vi "serialization test.vi"() -> (0 "no error":errorcluster, 1 "name ok":bool, 2 "serOK":bool, 3 "class identical":bool, 4 "keys ok":bool, 5 "version ok":bool)   [LabVIEW 2025, in "NISE_CEF_Tests.lvlib"]
uses:
  NISE_CEF_Tests.lvlib
  Trunk/Configuration Framework/serializable configuration/NISE_CEF_serializable configuration.lvclass
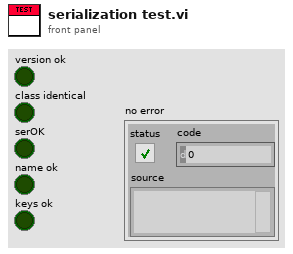
[diagram p1: front panel]
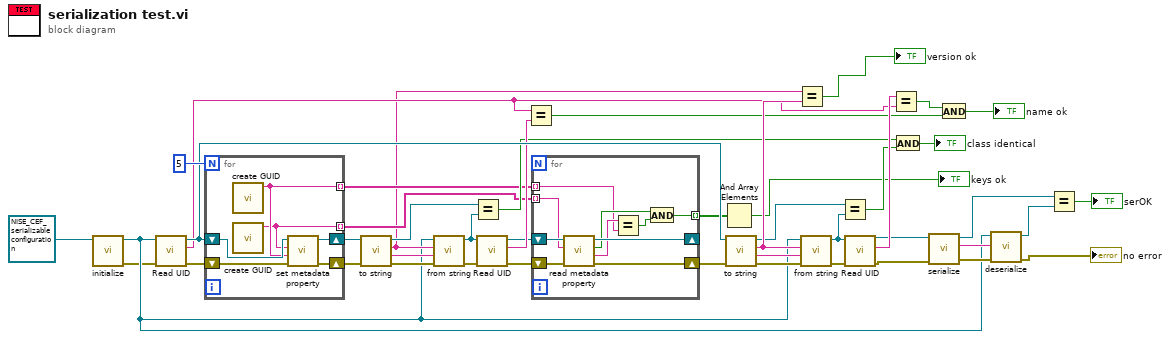
[diagram p0: block diagram]
diagram:
  n1 = call "initialize.vi"("configuration in"=refnum<class "NISE_CEF_serializable configuration.lvclass"> refnum ("configuration")) -> ("error out"=w1:errorcluster, "configuration out"=w2:refnum<class "NISE_CEF_serializable configuration.lvclass">)  [unwired: 8 in, 1 out]
  n2 = call "Read UID.vi"("error in"=w1, "configuration in"=w2) -> ("error out"=w38:errorcluster, "instance id"=w30:string, "configuration out"=w39:refnum<class "NISE_CEF_serializable configuration.lvclass">)  [unwired: 7 in]
  n3 = for {
    N: 5 -> [_]
    shift-right: [w50] -> w29
    shift-left: w39 -> [w51]
    shift-right: [w49] -> w35
    shift-left: w38 -> [w48]
    tunnel: [w47] -> w19 mode=indexing
    tunnel: [w46] -> w20 mode=indexing
    n4 = call "create GUID.vi"() -> ("uuid"=w47:string)  [unwired: 10 in, 1 out]
    n5 = call "create GUID.vi"() -> ("uuid"=w46:string)  [unwired: 10 in, 1 out]
    n6 = call "set metadata property.vi"("error in"=w48, "value"=w47, "key"=w46, "configuration in"=w51) -> ("error out"=w49:errorcluster, "configuration out"=w50:refnum<class "NISE_CEF_serializable configuration.lvclass">)  [unwired: 6 in]
  }
  n7 = call-dynamic "to string.vi"("error in"=w35, "configuration in"=w29) -> ("error out"=w36:errorcluster, "data"=w37:string, "version"=w4:string, "configuration out"=w26:refnum<class "NISE_CEF_serializable configuration.lvclass">)  [unwired: 6 in]
  n8 = call-dynamic "from string.vi"("error in"=w36, "data"=w37, "version"=w4, "configuration in"=w2) -> ("error out"=w32:errorcluster, "configuration out"=w28:refnum<class "NISE_CEF_serializable configuration.lvclass">)  [unwired: 6 in]
  n9 = Equal?(x=w26, y=w28) -> (x = y?=w21:bool)
  n10 = call "Read UID.vi"("error in"=w32, "configuration in"=w28) -> ("error out"=w17:errorcluster, "instance id"=w31:string, "configuration out"=w18:refnum<class "NISE_CEF_serializable configuration.lvclass">)  [unwired: 7 in]
  n11 = Equal?(x=w30, y=w31) -> (x = y?=w24:bool)
  n12 = for {
    tunnel: w20 -> [w57] mode=indexing
    tunnel: w19 -> [w54] mode=indexing
    shift-right: [w59] -> _
    shift-left: w18 -> [w60]
    shift-right: [w58] -> w16
    shift-left: w17 -> [w61]
    tunnel: [w52] -> w15 mode=indexing
    n13 = call "read metadata property.vi"("error in"=w61, "key"=w57, "configuration in"=w60) -> ("error out"=w58:errorcluster, "value"=w55:string, "found"=w56:bool, "configuration out"=w59:refnum<class "NISE_CEF_serializable configuration.lvclass">)  [unwired: 5 in]
    n14 = Equal?(x=w55, y=w54) -> (x = y?=w53:bool)
    n15 = And(x=w56, y=w53) -> (x .and. y?=w52:bool)
  }
  n16 = And Array Elements(Boolean array=w15) -> (logical AND=→"keys ok":bool)
  n17 = call-dynamic "to string.vi"("error in"=w16, "configuration in"=w39) -> ("error out"=w45:errorcluster, "data"=w41:string, "version"=w44:string, "configuration out"=w27:refnum<class "NISE_CEF_serializable configuration.lvclass">)  [unwired: 6 in]
  n18 = Equal?(x=w4, y=w44) -> (x = y?=→"version ok":bool)
  n19 = call-dynamic "from string.vi"("error in"=w45, "data"=w41, "version"=w44, "configuration in"=w2) -> ("error out"=w43:errorcluster, "configuration out"=w25:refnum<class "NISE_CEF_serializable configuration.lvclass">)  [unwired: 6 in]
  n20 = Equal?(x=w27, y=w25) -> (x = y?=w22:bool)
  n21 = call "Read UID.vi"("error in"=w43, "configuration in"=w25) -> ("error out"=w10:errorcluster, "instance id"=w42:string, "configuration out"=w11:refnum<class "NISE_CEF_serializable configuration.lvclass">)  [unwired: 7 in]
  n22 = Equal?(x=w42, y=w30) -> (x = y?=w33:bool)
  n23 = And(x=w21, y=w22) -> (x .and. y?=→"class identical":bool)
  n24 = call "serialize.vi"("error in"=w10, "configuration in"=w11) -> ("error out"=w12:errorcluster, "serialized form"=w8:string, "configuration out"=w6:refnum<class "NISE_CEF_serializable configuration.lvclass">)  [unwired: 7 in]
  n25 = And(x=w33, y=w24) -> (x .and. y?=→"name ok":bool)
  n26 = call "deserialize.vi"("error in"=w12, "serialized form"=w8, "configuration in"=w2) -> ("error out"=→"no error":errorcluster, "configuration out"=w7:refnum<class "NISE_CEF_serializable configuration.lvclass">)  [unwired: 7 in]
  n27 = Equal?(x=w6, y=w7) -> (x = y?=→"serOK":bool)
